vi "OMAR.vi"() -> ()   [LabVIEW 2021]
panel:
  out "Array":string[](array[string])
  in  "stop":bool
  in  "Tab control":T1(tab)
  in  "?":bool
  in  "log in":bool
  in  "User Name":string
  in  "Password":string
  in  "Ground Track Track":bool
  in  "Determine Area":bool
  in  "Target determination":bool
  in  "Session Time":bool
  in  "Shadow and Light":bool
  in  "Satellite Position":bool
  in  "Track":bool
  in  "Orbiteal Elements":bool
  in  "Home":bool
  in  "Drop your path":path
  out "Satellite catalog number 2":string
  out "Inclination":string
  out "Right asciension of the ascending node":string
  out "Eccentricity":string
  out "Argument of perigee":string
  out "Mean anomaly":string
  out "Line number 2":string caption="Line number"
  out "Line number":string
  out "Satellite catalog number 1":string
  out "Last two digits Vof launch year":string
  out "Launch number of the year":string
  out "Epoch year":string
  out "Epoch day of year":string
  out "Classification":string caption="Line number"
  out "Piece of the launch":string
  out "Your TLE":string
  in  "?":bool
  in  "?":bool
  in  "Track Info":bool
  out "?":bool
  out "?":cluster{"X":dbl, "Y":dbl}[](graph)
  in  "?":bool
  out "Lat":dbl
  out "Long":i32
  out "V":string
  out "R":string
  in  "?":bool
  in  "?":bool
  in  "?":bool
  in  "?":bool
  in  "?":bool
  in  "?":bool
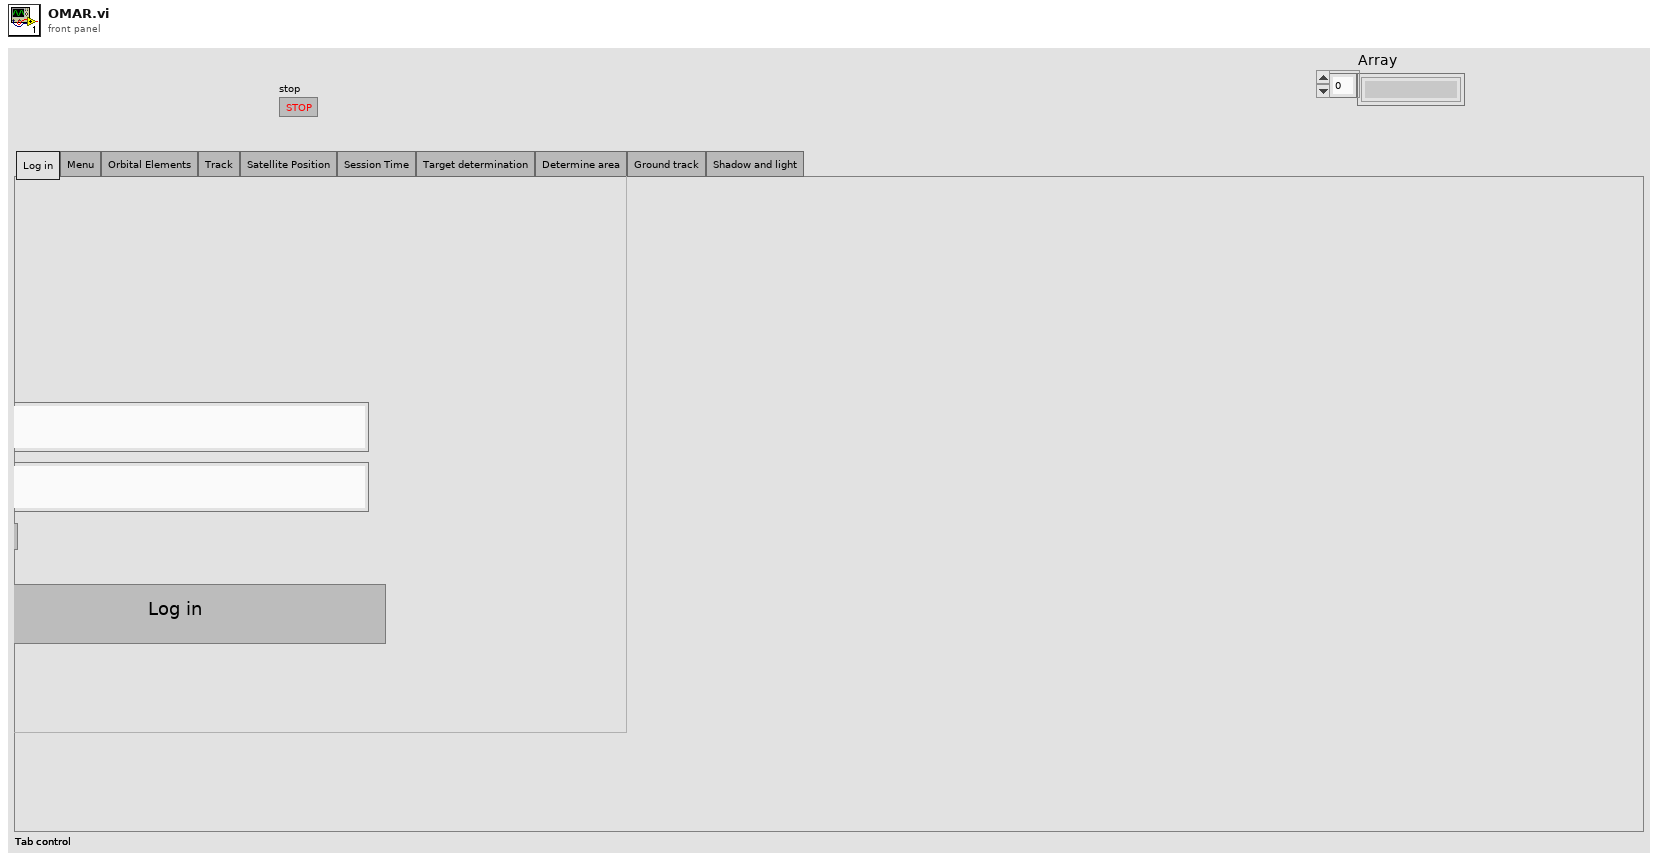
[diagram p1: front panel]
types:
  T1 = enum32{"Log in", "Menu", "Orbital Elements", "Track", "Satellite Position", "Session Time", "Target determination", "Determine area", "Ground track", "Shadow and light"}
  T2 = enum32{"Log in", "Menu", "Orbital Elements", "Track", "Satellite Position", "Session Time", "Target determination", "Determine area", "Ground track"}
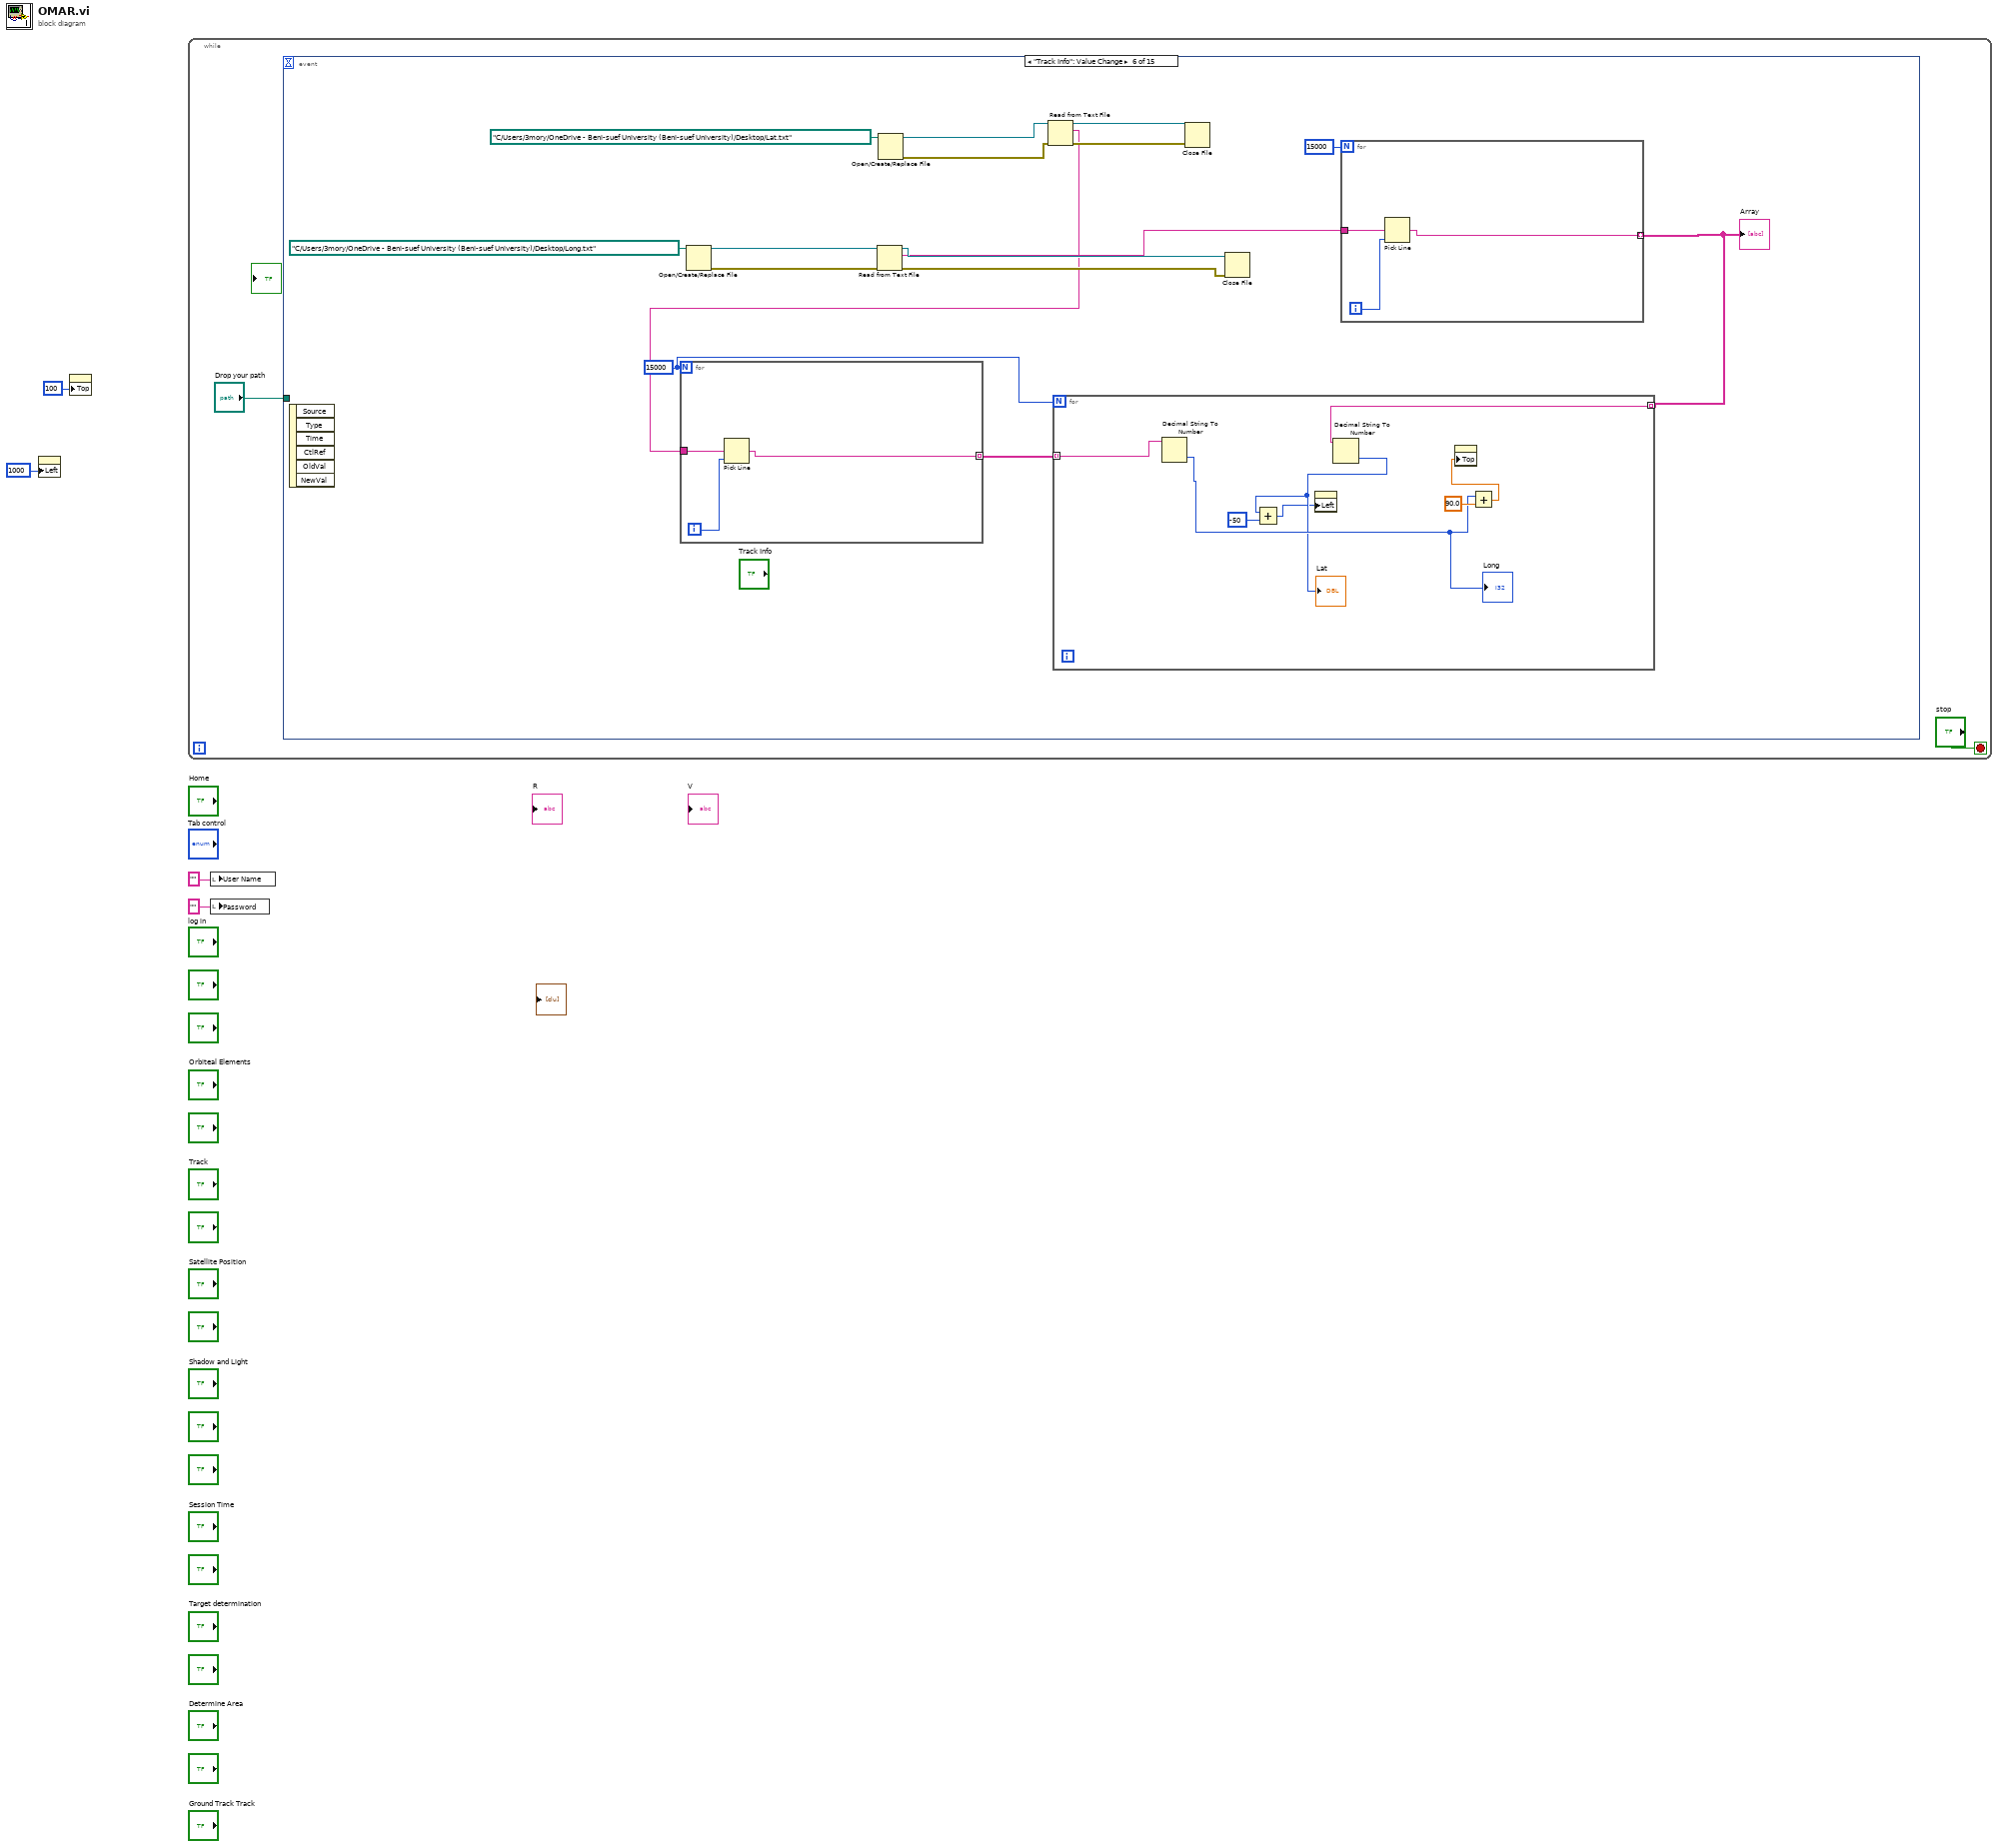
[diagram p0: block diagram]
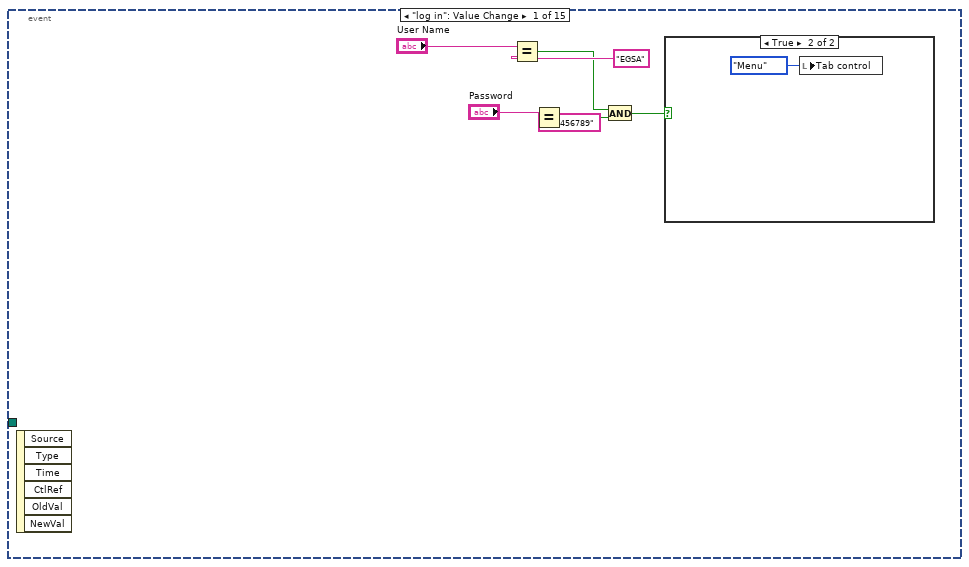
[diagram p2: hidden frame]
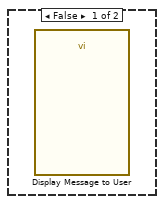
[diagram p3: hidden frame]
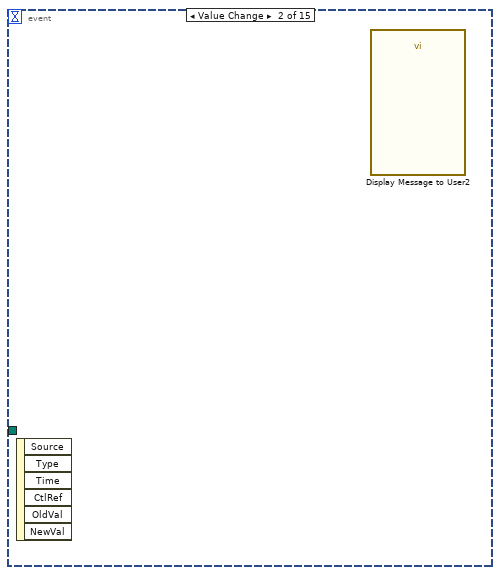
[diagram p4: hidden frame]
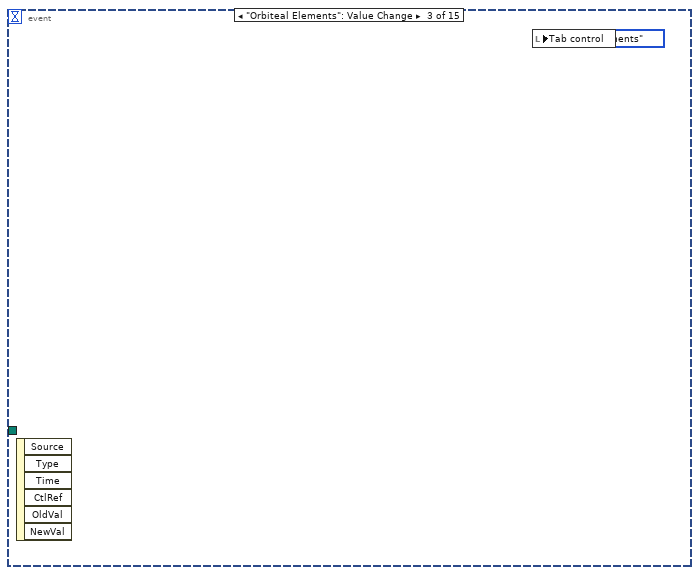
[diagram p5: hidden frame]
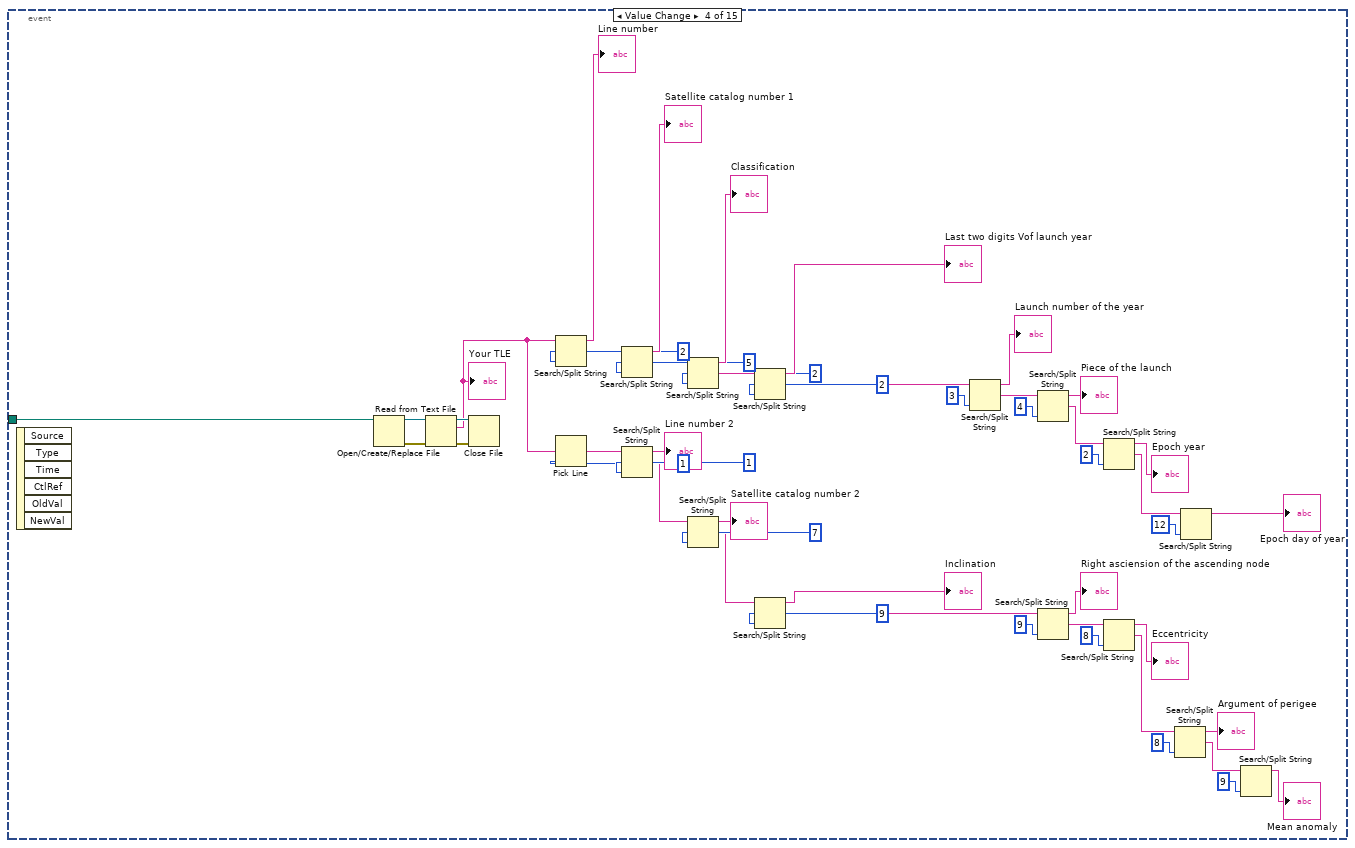
[diagram p6: hidden frame]
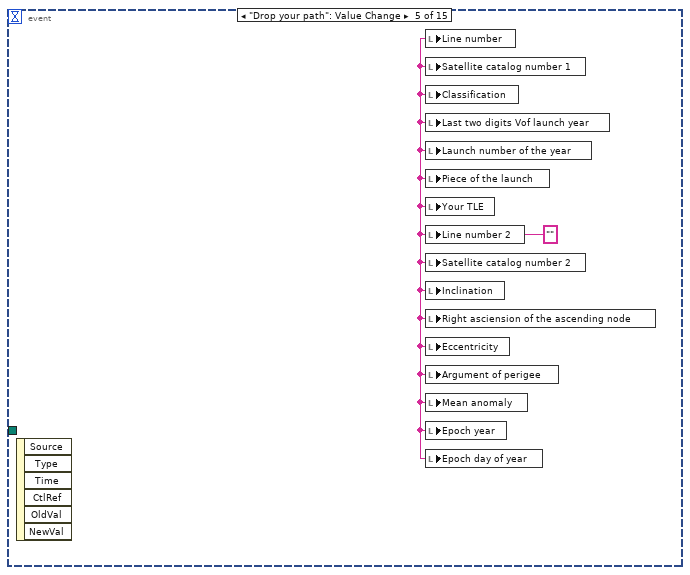
[diagram p7: hidden frame]
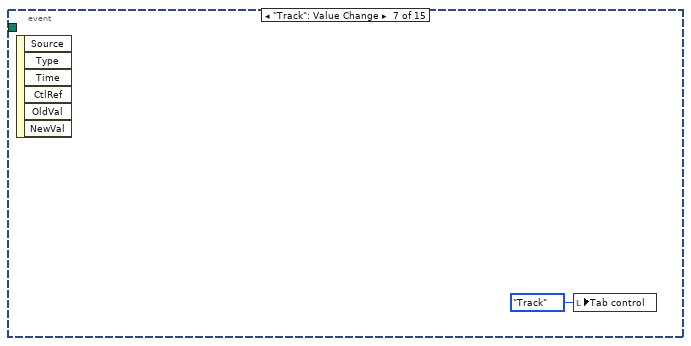
[diagram p8: hidden frame]
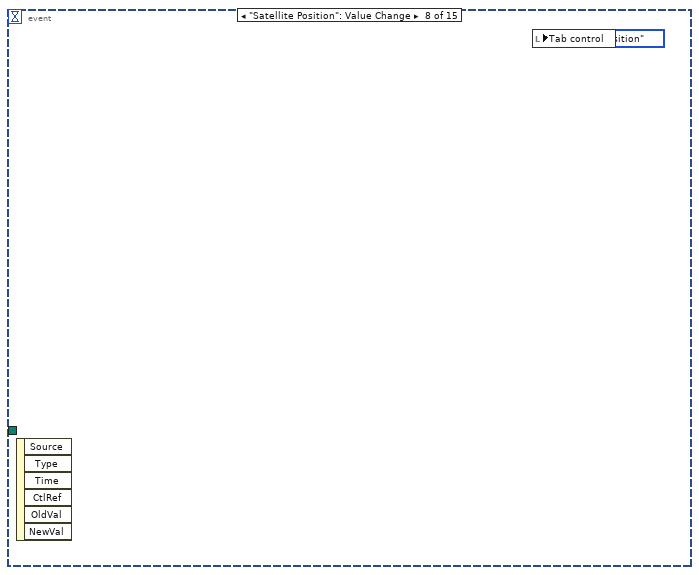
[diagram p9: hidden frame]
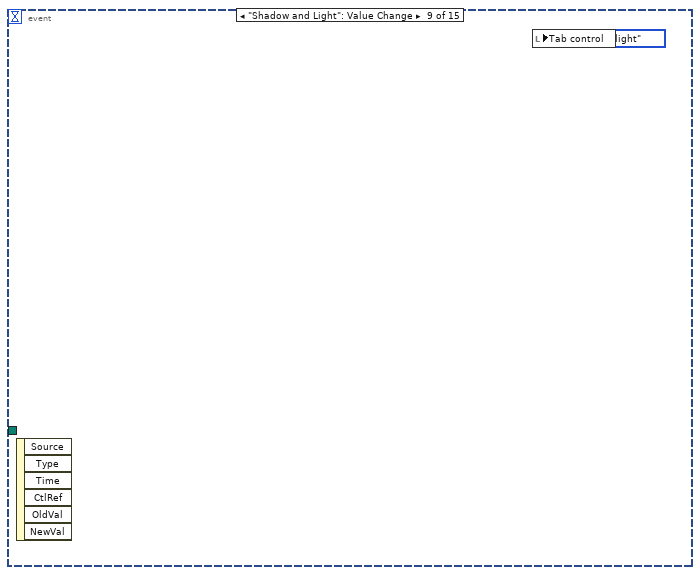
[diagram p10: hidden frame]
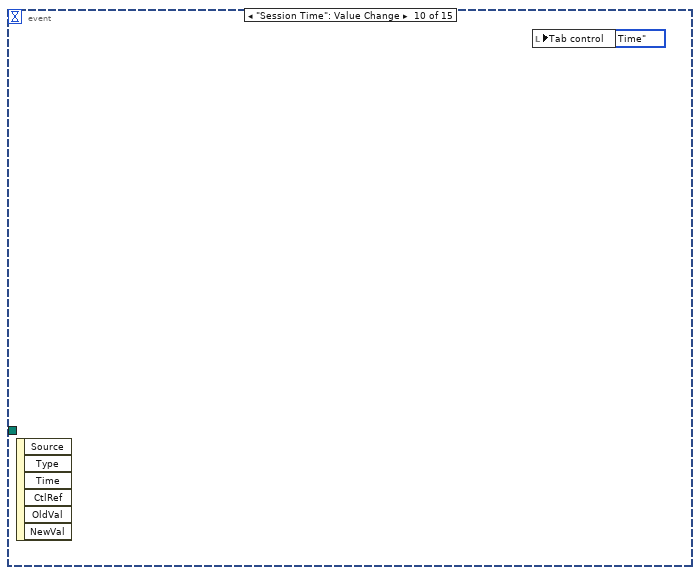
[diagram p11: hidden frame]
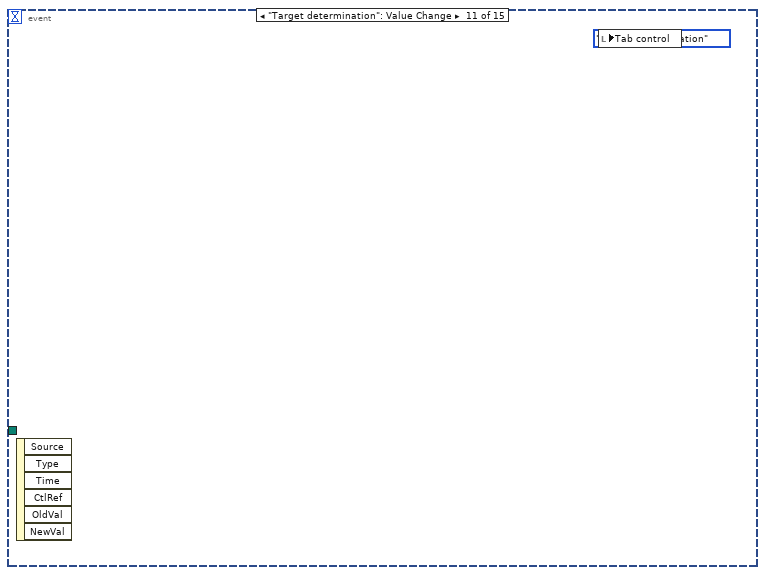
[diagram p12: hidden frame]
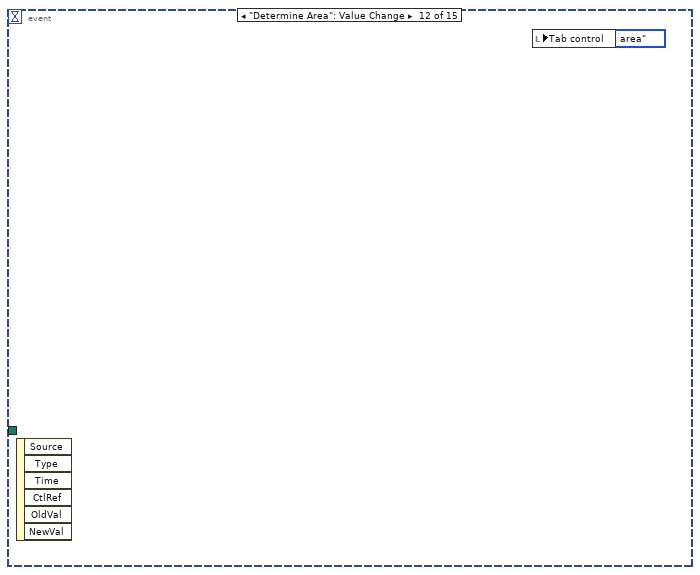
[diagram p13: hidden frame]
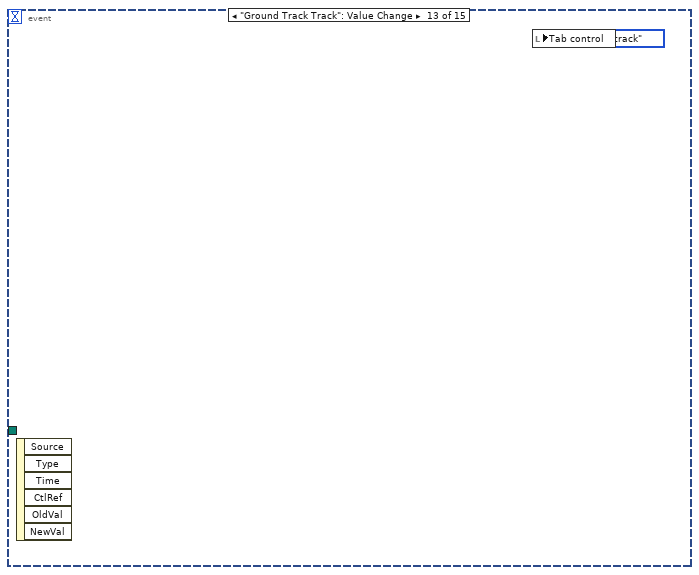
[diagram p14: hidden frame]
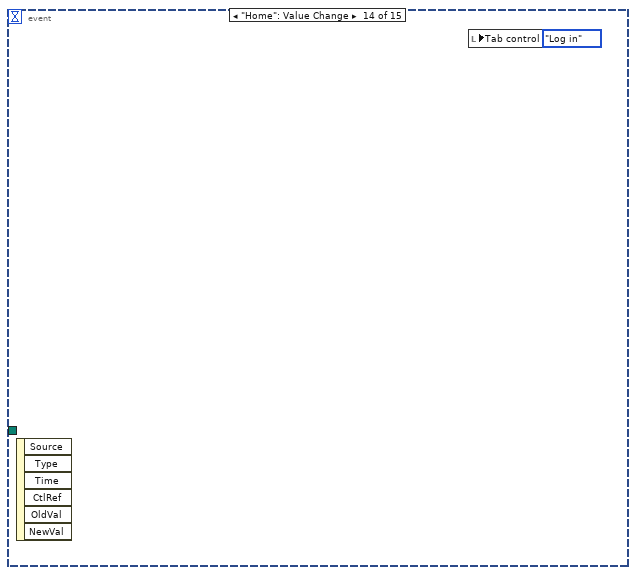
[diagram p15: hidden frame]
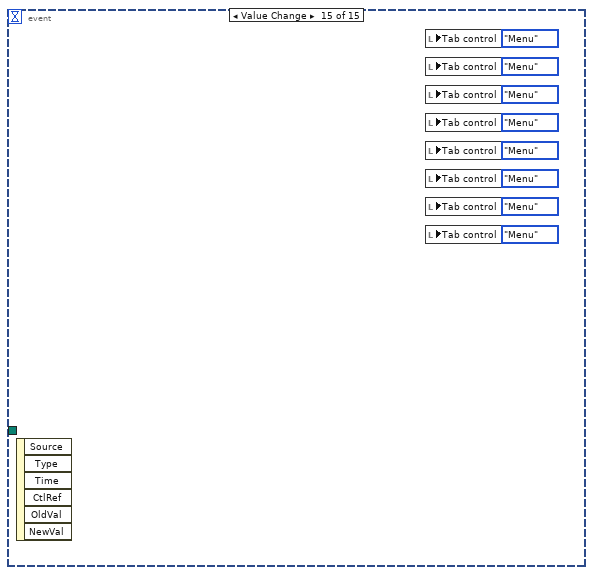
[diagram p16: hidden frame]
diagram:
  n1 = property class="Bool (strict)"("Left"=1000 ("Position:Left")) -> ()  [unwired: 2 in, 2 out]
  n2 = property class="Bool (strict)"("Top"=100 ("Position:Top")) -> ()  [unwired: 2 in, 2 out]
  n3 = while {
    stop <- "stop" stop-if-true
    n4 = event shown="[5] \"Track Info\": Value Change" {
      selector: _ -> [_ _ _ _ _ _ _ _ _ _ _ _ _ _ _]
      dyn-events: _ -> [_ _ _ _ _ _ _ _ _ _ _ _ _ _ _]
      timeout: _ -> [_ _ _ _ _ _ _ _ _ _ _ _ _ _ _]
      tunnel: "Drop your path" -> [_ _ _ w17 _ _ _ _ _ _ _ _ _ _ _]
      event "log in": Value Change {
        n5 = event-data() -> ()  [unwired: 1 in, 6 out]
        n6 = Equal?(x="User Name", y="EGSA") -> (x = y?=w8:bool)
        n7 = Equal?(x="Password", y="123456789") -> (x = y?=w9:bool)
        n8 = And(x=w8, y=w9) -> (x .and. y?=w7:bool)
        n9 = case shown="True" w7 {
          frame False {
            n10 = call "Display Message to User"() -> ()  [unwired: 10 in, 2 out]
          }
          frame True {
            n11 = local write "Tab control"(T1."Menu" ("Tab control")) -> ()
          }
        }
      }
      event Value Change {
        n12 = event-data() -> ()  [unwired: 1 in, 6 out]
        n13 = call "Display Message to User2"() -> ()  [unwired: 10 in, 2 out]
      }
      event "Orbiteal Elements": Value Change {
        n14 = event-data() -> ()  [unwired: 1 in, 6 out]
        n15 = local write "Tab control"(T1."Orbital Elements" ("Tab control")) -> ()
      }
      event Value Change {
        n16 = event-data() -> ()  [unwired: 1 in, 6 out]
        n17 = Open/Create/Replace File(file path (use dialog)=w17) -> (refnum out=w66:refnum<file>, error out=w65:errorcluster)  [unwired: 5 in, 1 out]
        n18 = Read from Text File(file (use dialog)=w66, error in=w65) -> (refnum out=w64:refnum<file>, text=w16:string, error out=w63:errorcluster)  [unwired: 2 in, 1 out]
        "Your TLE" <- w16
        n19 = Close File(refnum=w64, error in=w63) -> ()  [unwired: 2 out]
        n20 = Search/Split String(string=w16, offset (0)=2) -> (substring before match=→"Line number":string, match + rest of string=w33:string)  [unwired: 1 in, 1 out]
        n21 = Pick Line(multi-line string=w16, line index=1) -> (output string=w18:string)  [unwired: 1 in]
        n22 = Search/Split String(string=w33, offset (0)=5) -> (substring before match=→"Satellite catalog number 1":string, match + rest of string=w23:string)  [unwired: 1 in, 1 out]
        n23 = Search/Split String(string=w18, offset (0)=1) -> (substring before match=→"Line number 2":string, match + rest of string=w46:string)  [unwired: 1 in, 1 out]
        n24 = Search/Split String(string=w23, offset (0)=2) -> (substring before match=→"Classification":string, match + rest of string=w25:string)  [unwired: 1 in, 1 out]
        n25 = Search/Split String(string=w46, offset (0)=7) -> (substring before match=→"Satellite catalog number 2":string, match + rest of string=w44:string)  [unwired: 1 in, 1 out]
        n26 = Search/Split String(string=w25, offset (0)=2) -> (substring before match=→"Last two digits Vof launch year":string, match + rest of string=w30:string)  [unwired: 1 in, 1 out]
        n27 = Search/Split String(string=w44, offset (0)=9) -> (substring before match=→"Inclination":string, match + rest of string=w42:string)  [unwired: 1 in, 1 out]
        n28 = Search/Split String(string=w30, offset (0)=3) -> (substring before match=→"Launch number of the year":string, match + rest of string=w22:string)  [unwired: 1 in, 1 out]
        n29 = Search/Split String(string=w22, offset (0)=4) -> (substring before match=→"Piece of the launch":string, match + rest of string=w21:string)  [unwired: 1 in, 1 out]
        n30 = Search/Split String(string=w42, offset (0)=9) -> (substring before match=→"Right asciension of the ascending node":string, match + rest of string=w40:string)  [unwired: 1 in, 1 out]
        n31 = Search/Split String(string=w21, offset (0)=2) -> (substring before match=→"Epoch year":string, match + rest of string=w28:string)  [unwired: 1 in, 1 out]
        n32 = Search/Split String(string=w40, offset (0)=8) -> (substring before match=→"Eccentricity":string, match + rest of string=w38:string)  [unwired: 1 in, 1 out]
        n33 = Search/Split String(string=w38, offset (0)=8) -> (substring before match=→"Argument of perigee":string, match + rest of string=w36:string)  [unwired: 1 in, 1 out]
        n34 = Search/Split String(string=w28, offset (0)=12) -> (substring before match=→"Epoch day of year":string)  [unwired: 1 in, 2 out]
        n35 = Search/Split String(string=w36, offset (0)=9) -> (substring before match=→"Mean anomaly":string)  [unwired: 1 in, 2 out]
      }
      event "Drop your path": Value Change {
        w67 = "" ("Line number")
        n36 = event-data() -> ()  [unwired: 1 in, 6 out]
        n37 = local write "Line number"(w67) -> ()
        n38 = local write "Satellite catalog number 1"(w67) -> ()
        n39 = local write "Classification"(w67) -> ()
        n40 = local write "Last two digits Vof launch year"(w67) -> ()
        n41 = local write "Launch number of the year"(w67) -> ()
        n42 = local write "Piece of the launch"(w67) -> ()
        n43 = local write "Your TLE"(w67) -> ()
        n44 = local write "Line number 2"(w67) -> ()
        n45 = local write "Satellite catalog number 2"(w67) -> ()
        n46 = local write "Inclination"(w67) -> ()
        n47 = local write "Right asciension of the ascending node"(w67) -> ()
        n48 = local write "Eccentricity"(w67) -> ()
        n49 = local write "Argument of perigee"(w67) -> ()
        n50 = local write "Mean anomaly"(w67) -> ()
        n51 = local write "Epoch year"(w67) -> ()
        n52 = local write "Epoch day of year"(w67) -> ()
      }
      event "Track Info": Value Change {
        w68 = 15000
        n53 = event-data() -> ()  [unwired: 1 in, 6 out]
        n54 = Open/Create/Replace File(file path (use dialog)=path "C:/Users/3mory/OneDrive - Beni-suef University (Beni-suef University)/Desktop/Long.txt") -> (refnum out=w83:refnum<file>, error out=w82:errorcluster)  [unwired: 5 in, 1 out]
        n55 = Read from Text File(file (use dialog)=w83, error in=w82) -> (refnum out=w81:refnum<file>, text=w73:string, error out=w80:errorcluster)  [unwired: 2 in, 1 out]
        n56 = Open/Create/Replace File(file path (use dialog)=path "C:/Users/3mory/OneDrive - Beni-suef University (Beni-suef University)/Desktop/Lat.txt") -> (refnum out=w79:refnum<file>, error out=w78:errorcluster)  [unwired: 5 in, 1 out]
        n57 = Read from Text File(file (use dialog)=w79, error in=w78) -> (refnum out=w77:refnum<file>, text=w70:string, error out=w76:errorcluster)  [unwired: 2 in, 1 out]
        n58 = for {
          N: w68 -> [_]
          tunnel: w70 -> [w85]
          tunnel: [w84] -> w69 mode=indexing
          i -> [w86]
          n59 = Pick Line(multi-line string=w85, line index=w86) -> (output string=w84:string)  [unwired: 1 in]
        }
        n60 = Close File(refnum=w77, error in=w76) -> ()  [unwired: 2 out]
        n61 = Close File(refnum=w81, error in=w80) -> ()  [unwired: 2 out]
        n62 = for {
          N: 15000 -> [_]
          tunnel: w73 -> [w96]
          tunnel: [w95] -> w71 mode=indexing
          i -> [w97]
          n63 = Pick Line(multi-line string=w96, line index=w97) -> (output string=w95:string)  [unwired: 1 in]
        }
        "Array" <- w71
        n64 = for {
          N: w68 -> [_]
          tunnel: w71 -> [w94] mode=indexing
          tunnel: w69 -> [w93] mode=indexing
          n65 = Decimal String To Number(string=w93) -> (number=w91:i32)  [unwired: 2 in, 1 out]
          "Long" <- w91
          n66 = Decimal String To Number(string=w94) -> (number=w89:i32)  [unwired: 2 in, 1 out]
          "Lat" <- w89
          n67 = Add(x=w89, y=-50) -> (x+y=w87:i32)
          n68 = property class="Bool (strict)"("Left"=w87) -> ()  [unwired: 2 in, 2 out]
          n69 = Add(x=w91, y=90.0) -> (x+y=w90:dbl)
          n70 = property class="Bool (strict)"("Top"=w90) -> ()  [unwired: 2 in, 2 out]
        }
      }
      event "Track": Value Change {
        n71 = event-data() -> ()  [unwired: 1 in, 6 out]
        n72 = local write "Tab control"(T1."Track" ("Tab control")) -> ()
      }
      event "Satellite Position": Value Change {
        n73 = event-data() -> ()  [unwired: 1 in, 6 out]
        n74 = local write "Tab control"(T2."Satellite Position" ("Tab control")) -> ()
      }
      event "Shadow and Light": Value Change {
        n75 = event-data() -> ()  [unwired: 1 in, 6 out]
        n76 = local write "Tab control"(T1."Shadow and light" ("Tab control")) -> ()
      }
      event "Session Time": Value Change {
        n77 = event-data() -> ()  [unwired: 1 in, 6 out]
        n78 = local write "Tab control"(T1."Session Time" ("Tab control")) -> ()
      }
      event "Target determination": Value Change {
        n79 = event-data() -> ()  [unwired: 1 in, 6 out]
        n80 = local write "Tab control"(T1."Target determination" ("Tab control")) -> ()
      }
      event "Determine Area": Value Change {
        n81 = event-data() -> ()  [unwired: 1 in, 6 out]
        n82 = local write "Tab control"(T1."Determine area" ("Tab control")) -> ()
      }
      event "Ground Track Track": Value Change {
        n83 = event-data() -> ()  [unwired: 1 in, 6 out]
        n84 = local write "Tab control"(T1."Ground track" ("Tab control")) -> ()
      }
      event "Home": Value Change {
        n85 = event-data() -> ()  [unwired: 1 in, 6 out]
        n86 = local write "Tab control"(T1."Log in" ("Tab control")) -> ()
      }
      event Value Change {
        n87 = event-data() -> ()  [unwired: 1 in, 6 out]
        n88 = local write "Tab control"(T1."Menu" ("Tab control")) -> ()
        n89 = local write "Tab control"(T1."Menu" ("Tab control")) -> ()
        n90 = local write "Tab control"(T1."Menu" ("Tab control")) -> ()
        n91 = local write "Tab control"(T1."Menu" ("Tab control")) -> ()
        n92 = local write "Tab control"(T1."Menu" ("Tab control")) -> ()
        n93 = local write "Tab control"(T1."Menu" ("Tab control")) -> ()
        n94 = local write "Tab control"(T1."Menu" ("Tab control")) -> ()
        n95 = local write "Tab control"(T1."Menu" ("Tab control")) -> ()
      }
    }
  }
  n96 = local write "User Name"("" ("User Name")) -> ()
  n97 = local write "Password"("" ("Password")) -> ()
